vi "Main.vi"() -> ()   [LabVIEW 2016]
doc: "The myRIO Project template acquires acceleration data from the onboard accelerometer and displays the changes of acceleration values in a waveform chart."
uses:
  <vilib>/myRIO/Instrument Drivers/Onboard IO/PWM/typedefs/PWM Reference.ctl
  <vilib>/myRIO/Common/Instrument Driver Framework/Utilities/typedefs/myRIO Generic Hardware Reference.ctl
  <vilib>/myRIO/Common/Instrument Driver Framework/Utilities/typedefs/Hardware Version Enum.ctl
  <vilib>/myRIO/Common/Instrument Driver Framework/Utilities/typedefs/myRIO v1.0 Reference.ctl
  <vilib>/myRIO/Common/Instrument Driver Framework/Utilities/typedefs/Generic FPGA Reference.ctl
  <vilib>/myRIO/Common/Instrument Driver Framework/myRIO v1.0/PWM/typedefs/PWM Channels Enum.ctl
  <vilib>/myRIO/Instrument Drivers/Onboard IO/PWM/typedefs/PWM Configuration.ctl
  <vilib>/userdefined/High Color/nirio_resource_hc.ctl
  <vilib>/myRIO/Instrument Drivers/Onboard IO/DIO/typedefs/DIO Reference.ctl
  <vilib>/myRIO/Common/Instrument Driver Framework/myRIO v1.0/DIO/typedefs/DIO Channels List.ctl
  <vilib>/myRIO/Common/Instrument Driver Framework/myRIO v1.0/DIO/typedefs/DIO Channels Enum.ctl
  <vilib>/myRIO/Common/Instrument Driver Framework/myRIO v1.0/PWM/vis/myRIO v1.1 Open PWM.vi
  <vilib>/myRIO/Common/Instrument Driver Framework/Utilities/vis/Is FPGA Ref Available.vi
  <vilib>/myRIO/Common/Instrument Driver Framework/myRIO v1.0/DIO/vis/myRIO v1.1 Open DIO.vi
  <vilib>/myRIO/Instrument Drivers/Onboard IO/DIO/vis/Read.vi
  <vilib>/myRIO/Common/Instrument Driver Framework/Utilities/vis/Validate Channels.vi
  <vilib>/myRIO/Common/Instrument Driver Framework/myRIO v1.0/PWM/vis/myRIO v1.0 Reserve PWM.vi
  <vilib>/myRIO/Common/Instrument Driver Framework/myRIO v1.0/DIO/vis/myRIO v1.0 Reserve DIO.vi
  <vilib>/myRIO/Common/Instrument Driver Framework/myRIO v1.0/UART/vis/myRIO v1.0 Close UART.vi
  <vilib>/myRIO/Common/Instrument Driver Framework/myRIO v1.0/PWM/vis/myRIO v1.0 Build MUX Configuration PWM.vi
  <vilib>/myRIO/Common/Instrument Driver Framework/myRIO v1.0/Resource Manager/vis/myRIO v1.0 Reserve Channel List.vi
  <vilib>/myRIO/Common/Instrument Driver Framework/myRIO v1.0/DIO/vis/myRIO v1.0 Build MUX Configuration DIO.vi
  <vilib>/myRIO/Common/Instrument Driver Framework/myRIO v1.0/Resource Manager/vis/myRIO v1.0 Create Configuration List.vi
  <vilib>/myRIO/Common/Instrument Driver Framework/myRIO v1.0/Resource Manager/vis/myRIO v1.0 Reserve Channel.vi
  <vilib>/myRIO/Common/Instrument Driver Framework/myRIO v1.0/Resource Manager/vis/myRIO v1.0 Unreserve Channel.vi
  <vilib>/myRIO/Common/Instrument Driver Framework/myRIO v1.0/Resource Manager/vis/myRIO v1.0 Build Mutex Name.vi
  <vilib>/Utility/VariantDataType/GetNumericInfo.vi
  <vilib>/Utility/error.llb/Error Cluster From Error Code.vi
  <vilib>/myRIO/Common/Instrument Driver Framework/myRIO v1.0/myRIO v1.1 Open.vi
  <vilib>/myRIO/Common/Instrument Driver Framework/Utilities/vis/IO Manager.vi
  <vilib>/myRIO/Common/Instrument Driver Framework/Utilities/vis/Configuration Manager.vi
  <vilib>/myRIO/Common/Instrument Driver Framework/myRIO v1.0/Resource Manager/vis/myRIO v1.0 Configure IO.vi
  <vilib>/myRIO/Common/Instrument Driver Framework/myRIO v1.0/myRIO v1.0 Close.vi
  <vilib>/myRIO/Common/Instrument Driver Framework/myRIO v1.0/DIO/vis/myRIO v1.0 Read DIO.vi
  <vilib>/addons/control/pid/pid.llb/PID (DBL).vi
  <vilib>/myRIO/Common/Instrument Driver Framework/myRIO v1.0/PWM/vis/myRIO v1.0 Write PWM.vi
  <vilib>/myRIO/Common/Instrument Driver Framework/Utilities/vis/FPGA Ref Manager.vi
  <vilib>/myRIO/Common/Instrument Driver Framework/myRIO v1.0/myRIO v1.0 Reset FPGA.vi
  <vilib>/myRIO/Common/Instrument Driver Framework/myRIO v1.0/IRQ/vis/myRIO v1.0 IRQ Info FGV.vi
  <vilib>/myRIO/Common/Instrument Driver Framework/myRIO v1.0/IRQ/vis/myRIO v1.0 Timer IRQ Info FGV.vi
  <vilib>/myRIO/Common/Instrument Driver Framework/myRIO v1.0/IRQ/vis/myRIO v1.0 ISR Agent.vi
  <vilib>/myRIO/Instrument Drivers/Onboard IO/PWM/vis/myRIO PWM Open.xnode
  <vilib>/myRIO/Express VI/Onboard IO/DI/DI Express VI.xnode
  <vilib>/myRIO/Instrument Drivers/Onboard IO/DIO/vis/myRIO DIO Open.xnode
  <vilib>/myRIO/Instrument Drivers/Onboard IO/DIO/DIO.lvlib
  <vilib>/myRIO/Instrument Drivers/Onboard IO/PWM/PWM.lvlib
  <vilib>/myRIO/Instrument Drivers/Utilities/Utilities.lvlib
  <vilib>/addons/control/pid/NI_PID_pid.lvlib
panel:
  in  "Korrektur":dbl
  out "output":dbl format="%.2f"
  out "A/DIO7 (Pin 25)":bool
  out "A/DIO6 (Pin 23)":bool
  out "A/DIO5 (Pin 21)":bool
  out "A/DIO4 (Pin 19)":bool
  out "A/DIO3 (Pin 17)":bool
  out "A/DIO2 (Pin 15)":bool
  out "A/DIO1 (Pin 13)":bool
  out "A/DIO0 (Pin 11)":bool
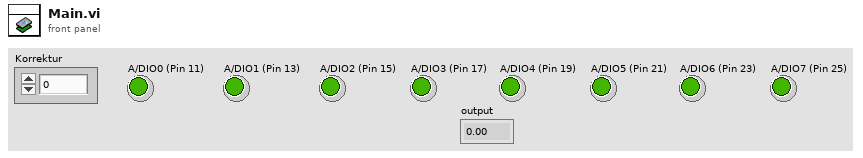
[diagram p1: front panel]
types:
  T1 = typedef "PWM.lvlib/PWM Reference.ctl" = cluster{"myRIO Reference":T2, "PWM Channels Enum":T6, "PWM Configuration":T7}
  T2 = typedef "myRIO Generic Hardware Reference.ctl" = cluster{"myRIO Model":T3, "myRIO Hardware Reference":T4}
  T3 = typedef "Hardware Version Enum.ctl" = enum16{"Unknown", "myRIO-1900", "myRIO-1950", "roboRIO", "NI ELVIS RIO CM"}
  T4 = typedef "myRIO v1.0 Reference.ctl" = cluster{"Generic FPGA Reference":T5, "Allow multiple opens":bool}
  T5 = typedef "Generic FPGA Reference.ctl" = refnum<k20>
  T6 = typedef "PWM Channels Enum.ctl" = enum16{"Not Connected", "C/PWM0", "C/PWM1", "A/PWM0", "A/PWM1", "A/PWM2", "B/PWM0", "B/PWM1", "B/PWM2", "PWM/PWM0", "PWM/PWM1", "PWM/PWM2", "PWM/PWM3", "PWM/PWM4", "PWM/PWM5", "PWM/PWM6", "PWM/PWM7", "PWM/PWM8", "PWM/PWM9"}
  T7 = typedef "PWM.lvlib/PWM Configuration.ctl" = cluster{"Frequency":dbl, "Duty Cycle":dbl}
  T8 = typedef "DIO.lvlib/DIO Reference.ctl" = cluster{"myRIO Reference":T2, "DIO Channels List":T9}
  T9 = typedef "DIO Channels List.ctl" = T10[]
  T10 = typedef "DIO Channels Enum.ctl" = enum16{"Not Connected", "C/DIO0", "C/DIO1", "C/DIO2", "C/DIO3", "C/DIO4", "C/DIO5", "C/DIO6", "C/DIO7", "A/DIO0", "A/DIO1", "A/DIO2", "A/DIO3", "A/DIO4", "A/DIO5", "A/DIO6", "A/DIO7", "A/DIO8", "A/DIO9", "A/DIO10", "A/DIO11", "A/DIO12", "A/DIO13", "A/DIO14", "A/DIO15", "B/DIO0", "B/DIO1", "B/DIO2", "B/DIO3", "B/DIO4", "B/DIO5", "B/DIO6", "B/DIO7", "B/DIO8", "B/DIO9", "B/DIO10", "B/DIO11", "B/DIO12", "B/DIO13", "B/DIO14", "B/DIO15", "LED0", "LED1", "LED2", "LED3", "Button0", "DIO/DIO0", "DIO/DIO1", "DIO/DIO2", "DIO/DIO3", "DIO/DIO4", "DIO/DIO5", "DIO/DIO6", "DIO/DIO7", "DIO/DIO8", "DIO/DIO9", "SPI/CS0", "SPI/CS1", "SPI/CS2", "SPI/CS3", "LED RADIO (Green)", "LED RADIO (Red)", "LED COMM (Green)", "LED COMM (Red)", "LED MODE (Green)", "LED MODE (Red)"}
  T11 = typedef "nirio_resource_hc.ctl" = tag
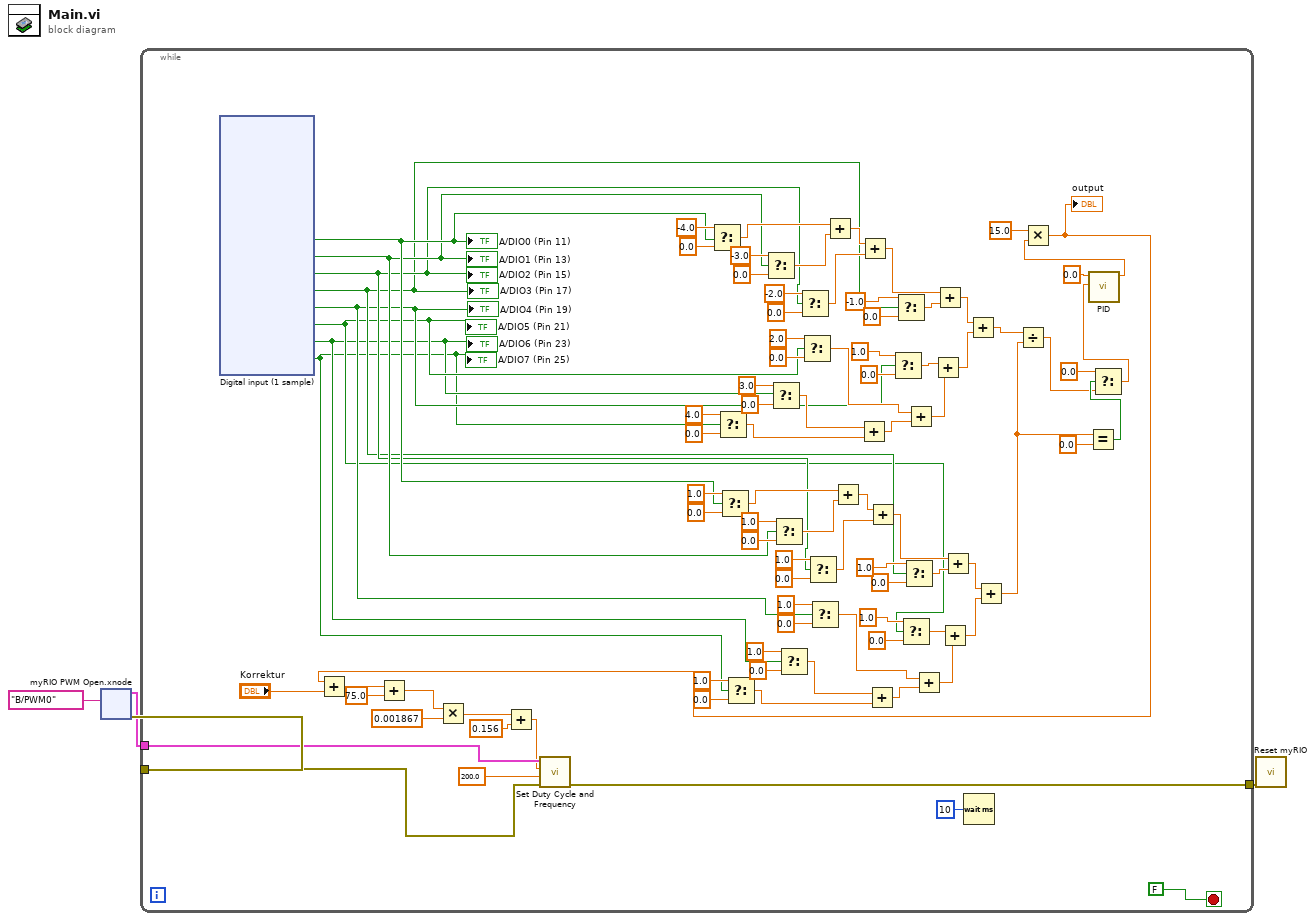
[diagram p0: block diagram]
diagram:
  n1 = xnode "myRIO PWM Open.xnode"("Channel Name"=tag "B/PWM0") -> ("error out"=w3:errorcluster, "PWM Ref Out"=w2:T1)  [unwired: 2 in]
  n2 = while {
    tunnel: w3 -> [w18]
    tunnel: w2 -> [w96]
    tunnel: [w95] -> w1
    stop <- FALSE stop-if-true
    n3 = xnode "Digital input (1 sample)"() -> ("A/DIO0 (Pin 11)"=w33:bool, "A/DIO1 (Pin 13)"=w32:bool, "A/DIO2 (Pin 15)"=w31:bool, "A/DIO3 (Pin 17)"=w30:bool, "A/DIO4 (Pin 19)"=w29:bool, "A/DIO5 (Pin 21)"=w28:bool, "A/DIO6 (Pin 23)"=w27:bool, "A/DIO7 (Pin 25)"=w26:bool)  [unwired: 1 in, 1 out]
    "A/DIO0 (Pin 11)" <- w33
    "A/DIO1 (Pin 13)" <- w32
    "A/DIO2 (Pin 15)" <- w31
    "A/DIO3 (Pin 17)" <- w30
    "A/DIO4 (Pin 19)" <- w29
    "A/DIO5 (Pin 21)" <- w28
    "A/DIO6 (Pin 23)" <- w27
    "A/DIO7 (Pin 25)" <- w26
    n4 = Select(t=-4.0, s=w33, f=0.0) -> (s? t:f=w83:dbl)
    n5 = Select(t=4.0, s=w26, f=0.0) -> (s? t:f=w75:dbl)
    n6 = Select(t=1.0, s=w33, f=0.0) -> (s? t:f=w53:dbl)
    n7 = Select(t=1.0, s=w26, f=0.0) -> (s? t:f=w45:dbl)
    n8 = Select(t=-3.0, s=w32, f=0.0) -> (s? t:f=w82:dbl)
    n9 = Select(t=3.0, s=w27, f=0.0) -> (s? t:f=w74:dbl)
    n10 = Select(t=1.0, s=w32, f=0.0) -> (s? t:f=w52:dbl)
    n11 = Select(t=1.0, s=w27, f=0.0) -> (s? t:f=w44:dbl)
    n12 = Select(t=-2.0, s=w31, f=0.0) -> (s? t:f=w80:dbl)
    n13 = Select(t=2.0, s=w28, f=0.0) -> (s? t:f=w72:dbl)
    n14 = Select(t=1.0, s=w31, f=0.0) -> (s? t:f=w50:dbl)
    n15 = Select(t=1.0, s=w29, f=0.0) -> (s? t:f=w42:dbl)
    n16 = Add(x=w83, y=w82) -> (x+y=w81:dbl)
    n17 = Add(x=w53, y=w52) -> (x+y=w51:dbl)
    n18 = Add(x=w74, y=w75) -> (x+y=w73:dbl)
    n19 = Add(x=w81, y=w80) -> (x+y=w77:dbl)
    n20 = Add(x=w44, y=w45) -> (x+y=w43:dbl)
    n21 = Add(x=w51, y=w50) -> (x+y=w47:dbl)
    n22 = Select(t=1.0, s=w29, f=0.0) -> (s? t:f=w70:dbl)
    n23 = Select(t=-1.0, s=w30, f=0.0) -> (s? t:f=w76:dbl)
    n24 = Select(t=1.0, s=w28, f=0.0) -> (s? t:f=w40:dbl)
    n25 = Select(t=1.0, s=w30, f=0.0) -> (s? t:f=w46:dbl)
    n26 = Add(x=w72, y=w73) -> (x+y=w71:dbl)
    n27 = Add(x=w42, y=w43) -> (x+y=w41:dbl)
    n28 = Add(x=w70, y=w71) -> (x+y=w64:dbl)
    n29 = Add(x=w77, y=w76) -> (x+y=w65:dbl)
    n30 = Add(x=w40, y=w41) -> (x+y=w34:dbl)
    n31 = Add(x=w47, y=w46) -> (x+y=w35:dbl)
    n32 = Wait (ms)(milliseconds to wait=u32 10) -> ()  [unwired: 1 out]
    n33 = Add(x=w65, y=w64) -> (x+y=w24:dbl)
    n34 = Add(x=w35, y=w34) -> (x+y=w23:dbl)
    n35 = Divide(x=w24, y=w23) -> (x/y=w19:dbl)
    n36 = Equal?(x=w23, y=0.0) -> (x = y?=w21:bool)
    n37 = Select(t=0.0, s=w21, f=w19) -> (s? t:f=w6:dbl)
    n38 = call-poly <vilib>:"PID.vi"("process variable"=w6, "setpoint"=0.0) -> ("output"=w5:dbl)  [unwired: 8 in, 1 out]
    n39 = Multiply(x=15.0, y=w5) -> (x*y=w7:dbl)
    "output" <- w7
    n40 = Add(x=w7, y="Korrektur") -> (x+y=w11:dbl)
    n41 = Add(x=w11, y=75.0) -> (x+y=w10:dbl)
    n42 = Multiply(x=w10, y=0.001867) -> (x*y=w15:dbl)
    n43 = Add(x=w15, y=0.156) -> (x+y=w13:dbl)
    n44 = call <vilib>:"Set Duty Cycle and Frequency.vi"("error in (no error)"=w18, "Frequency [Hz]"=200.0 ("y"), "Duty Cycle"=w13, "PWM Ref In"=w96) -> ("error out"=w95:errorcluster)  [unwired: 5 in, 1 out]
  }
  n45 = call <vilib>:"Reset myRIO.vi"("error in (no error)"=w1) -> ()  [unwired: 10 in, 1 out]
